vi "读取Start Time.vi"(8 "error in (no error)":errorcluster caption="错误输入（无错误）", 11 "Timer输入":refnum<class "Timer.lvclass">) -> (0 "error out":errorcluster caption="错误输出", 2 "Start Time":dbl, 3 "Timer输出":refnum<class "Timer.lvclass">)   [LabVIEW 2018, in "Timer.lvclass"]
uses:
  Timer.lvclass
  Timer.lvclass/Timer.ctl
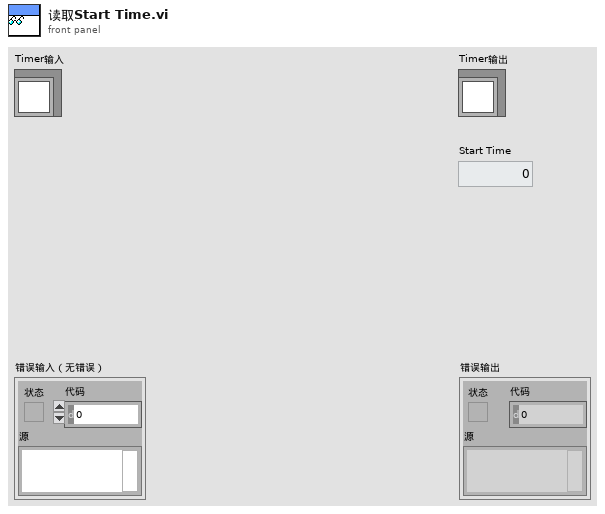
[diagram p1: front panel]
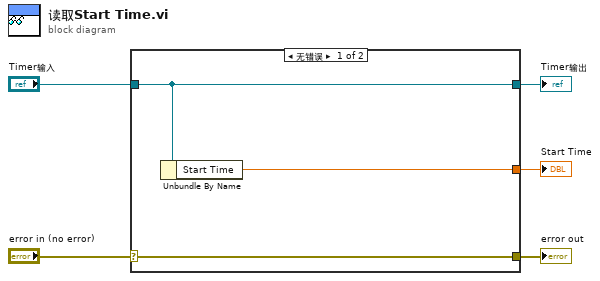
[diagram p0: block diagram]
diagram:
  n1 = case shown="无错误" "error in (no error)" {
    selector: "error in (no error)" -> [w8 w9]
    tunnel: [w8 w9] -> w4
    tunnel: [w7 w10] -> w2
    tunnel: "Timer输入" -> [w7 w10]
    tunnel: [w6 _] -> w1
    frame No Error {
      n2 = Unbundle By Name(w7) -> ("Start Time"=w6:dbl)
    }
    frame Error {
    }
  }
  "error out" <- w4
  "Timer输出" <- w2
  "Start Time" <- w1
